vi "RSZVB Set Trace Math State.vi"(8 "error in (no error)":errorcluster {"code" format="%.0x"}, 9 "Math State (F: Off)":bool, 10 "Channel (Trace) (1)":i32=1, 11 "VISA session":refnum<visa-resource-name>) -> (0 "error out":errorcluster {"code" format="%.0x"}, 3 "dup VISA session":refnum<visa-resource-name>)   [LabVIEW 2011]
doc: "This VI activates or deactivates the mathematical mode where the mathematical trace defined via CALCulate<Ch/Tr>:MATH[:EXPRession]:SDEFine is calculated and displayed instead of the active data trace.\n\nNote(s):\n\nThis VI is not valid for mathematical traces calculated via CALCulate<Ch/Tr>:MATH:FUNCtion.\n\nRemote-control command(s):\nCALCulate<Ch/Tr>:MATH:STATe <Boolean>"
panel:
  # "On\nOff"
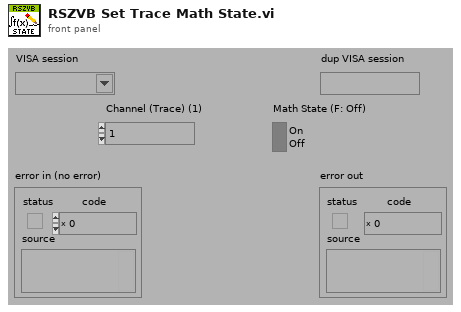
[diagram p1: front panel]
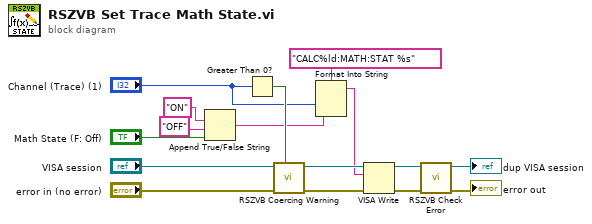
[diagram p0: block diagram]
diagram:
  n1 = Append True/False String(1:"Math State (F: Off)", 2:"OFF", 3:"ON") -> (0:w1:string)  [unwired: 1 in]
  n2 = Greater Than 0?(x="Channel (Trace) (1)") -> (x > 0?=w8:bool)
  n3 = call "RSZVB Coercing Warning.vi"("In Range?"=w8, "error in (no error)"="error in (no error)", "VISA session"="VISA session") -> ("error out"=w12:errorcluster, "dup VISA session"=w13:refnum<visa-resource-name>)  [unwired: 7 in]
  n4 = Format Into String(format string="CALC%ld:MATH:STAT %s", "Channel (Trace) (1)", w1) -> (resulting string=w9:string)  [unwired: 2 in, 1 out]
  n5 = VISA Write(VISA resource name=w13, write buffer=w9, error in (no error)=w12) -> (VISA resource name out=w10:refnum<visa-resource-name>, error out=w11:errorcluster)  [unwired: 1 out]
  n6 = call "RSZVB Check Error.vi"("error in (no error)"=w11, "VISA session"=w10) -> ("error out"=→"error out":errorcluster, "dup VISA session"=→"dup VISA session":refnum<visa-resource-name>)  [unwired: 8 in]
